vi "Create Special Complex Matrix.vi"(0 "matrix type":i32(ring) items=["Identity", "Diagonal", "Toeplitz", "Vandermonde", "Companion", "Hankel", "Hadamard", "Wilkinson", "Hilbert", "Inverse Hilbert", "Rosser", "Pascal"], 1 "matrix size":i32, 3 "Input Vector1":cdb[](array[numeric]) format="%.2f", 4 "Input Vector2":cdb[](array[numeric]) format="%.2f") -> (5 "Special Matrix":T1, 6 "error":i32)   [LabVIEW 2018, in "NI_AALPro.lvlib"]
doc: "Generates a special matrix based on <B>matrix type</B>. The data types you wire to the <B>Input Vector2</B> and <B>Input Vector1</B> inputs determine the polymorphic instance to use."
uses:
  <vilib>/Analysis/NI_AALPro.lvlib
  ComplexMatrix.ctl
  NI_Matrix.lvlib
  <resource>/lvanlys.dll
panel:
  # "Create Special Complex Matrix"
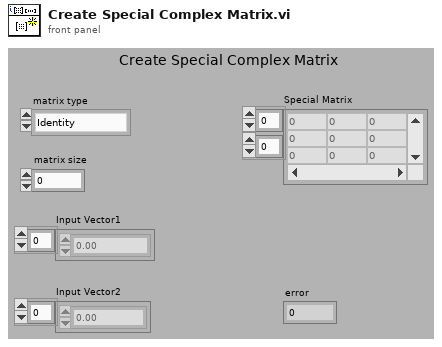
[diagram p1: front panel]
types:
  T1 = typedef "NI_Matrix.lvlib/ComplexMatrix.ctl" = cdb[][]
  T2 = typedef "NI_Matrix.lvlib/RealMatrix.ctl" = dbl[][]
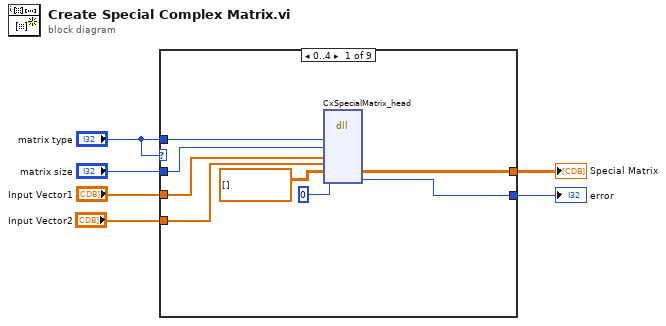
[diagram p0: block diagram]
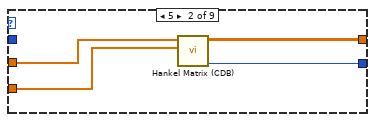
[diagram p2: hidden frame]
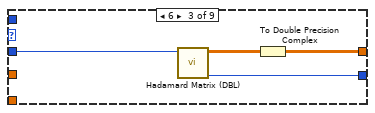
[diagram p3: hidden frame]
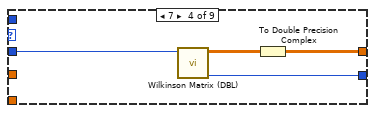
[diagram p4: hidden frame]
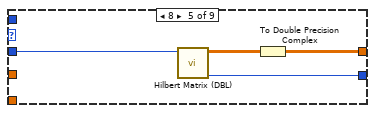
[diagram p5: hidden frame]
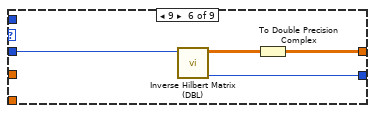
[diagram p6: hidden frame]
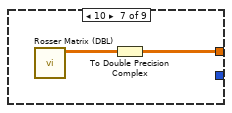
[diagram p7: hidden frame]
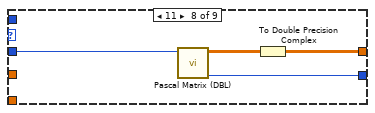
[diagram p8: hidden frame]
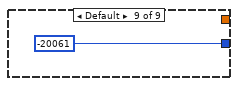
[diagram p9: hidden frame]
diagram:
  n1 = case shown="0..4" "matrix type" {
    tunnel: "matrix type" -> [w12 _ _ _ _ _ _ _ _]
    tunnel: "matrix size" -> [w11 _ w21 w25 w29 w32 _ w38 _]
    tunnel: "Input Vector1" -> [w10 w17 _ _ _ _ _ _ _]
    tunnel: [w8 w15 w19 w23 w27 w31 w35 w37 _] -> w2
    tunnel: [w7 w18 w22 w26 w30 w33 _ w39 -20061] -> w1
    tunnel: "Input Vector2" -> [w9 w16 _ _ _ _ _ _ _]
    frame 0..4 {
      n2 = dll-call lib="C:/Program Files (x86)/National Instruments/LabVIEW 2018/resource/lvanlys.*" fn="CxSpecialMatrix_head"("matrix type"=w12, "matrix size"=w11, "Input Vector1"=w10, "Input Vector2"=w9, "Special Matrix"=T1 [], 0) -> ("Special Matrix"=w8:T1, w7:i32)  [unwired: 8 in, 2 out]
    }
    frame 5 {
      n3 = call "Hankel Matrix (CDB).vi"("Input Vector2"=w16, "Input Vector1"=w17) -> ("error"=w18:i32, "Hankel Matrix"=w15:T1)  [unwired: 8 in]
    }
    frame 6 {
      n4 = call "Hadamard Matrix (DBL).vi"("matrix size"=w21) -> ("error"=w22:i32, "Hadamard Matrix"=w20:T2)  [unwired: 9 in]
      n5 = To Double Precision Complex(1:w20) -> (0:w19:cdb[][])
    }
    frame 7 {
      n6 = call "Wilkinson Matrix (DBL).vi"("matrix size"=w25) -> ("error"=w26:i32, "Wilkinson Matrix"=w24:T2)  [unwired: 9 in]
      n7 = To Double Precision Complex(1:w24) -> (0:w23:cdb[][])
    }
    frame 8 {
      n8 = call "Hilbert Matrix (DBL).vi"("matrix size"=w29) -> ("error"=w30:i32, "Hilbert Matrix"=w28:T2)  [unwired: 9 in]
      n9 = To Double Precision Complex(1:w28) -> (0:w27:cdb[][])
    }
    frame 9 {
      n10 = call "Inverse Hilbert Matrix (DBL).vi"("matrix size"=w32) -> ("error"=w33:i32, "Inverse Hilbert Matrix"=w34:T2)  [unwired: 9 in]
      n11 = To Double Precision Complex(1:w34) -> (0:w31:cdb[][])
    }
    frame 10 {
      n12 = call "Rosser Matrix (DBL).vi"() -> ("Rosser Matrix"=w36:T2)  [unwired: 11 in]
      n13 = To Double Precision Complex(1:w36) -> (0:w35:cdb[][])
    }
    frame 11 {
      n14 = call "Pascal Matrix (DBL).vi"("matrix size"=w38) -> ("error"=w39:i32, "Pascal Matrix"=w40:T2)  [unwired: 9 in]
      n15 = To Double Precision Complex(1:w40) -> (0:w37:cdb[][])
    }
    frame Default {
    }
  }
  "Special Matrix" <- w2
  "error" <- w1
